vi "Launcher.vi"() -> ()   [LabVIEW 2018]
uses:
  MQTT_Server_Actor/MQTT_Server_Actor.lvclass
  D:/Program Files (x86)/National Instruments/LabVIEW 2018/vi.lib/ActorFramework/Actor/Actor.lvclass
  MQTT_Client_Actor.lvclass
  CreateClient.ctl
  <vilib>/ActorFramework/Actor/Actor.lvclass
  MQTT_Server_Actor Messages/1_StartStopServer Msg/1_StartStopServer Msg.lvclass
  MQTT_Client_Actor Messages/1_CreateClient Msg/1_CreateClient Msg.lvclass
panel:
  in  "ClientNO.":i32=2
  in  "ServerNO.":i32=1
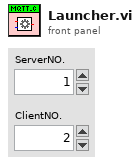
[diagram p1: front panel]
types:
  T1 = typedef "MQTT_Client_Actor.lvlib/MQTT_Client_Actor.lvclass/CreateClient.ctl" = cluster{"address":string, "port":u16, "UserName":string, "Pwd":string}
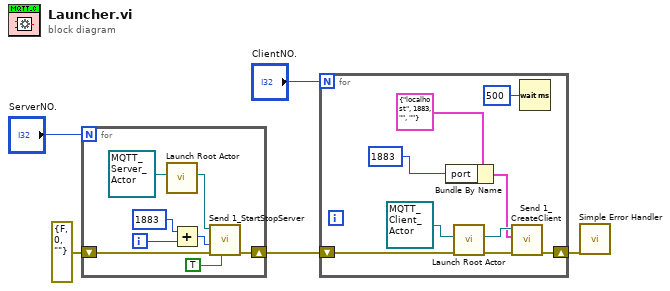
[diagram p0: block diagram]
diagram:
  n1 = for {
    N: "ServerNO." -> [_]
    shift-right: [w8] -> w3
    shift-left: errorcluster {"status"=FALSE, "code"=0, "source"=""} ("error out") -> [w7]
    i -> [w10]
    n2 = call <vilib>:"Launch Root Actor.vi"("Actor"=refnum<class "MQTT_Server_Actor.lvclass"> refnum ("MQTT_Server_Actor.lvlib:MQTT_Server_Actor.lvclass")) -> ("Actor's Enqueuer"=w12:refnum<class "Message Enqueuer.lvclass">)  [unwired: 9 in, 1 out]
    n3 = Add(x=u16 1883 ("remote port (80)"), y=w10) -> (x+y=w9:i32)
    n4 = call "Send 1_StartStopServer.vi"("T:start"=TRUE, "error in (no error)"=w7, "remote port (80)"=w9, "Message Enqueuer in"=w12) -> ("error out"=w8:errorcluster)  [unwired: 6 in, 1 out]
  }
  n5 = for {
    N: "ClientNO." -> [_]
    shift-right: [w15] -> w1
    shift-left: w3 -> [w17]
    n6 = Bundle By Name(cluster=T1 {"address"="localhost", "port"=1883, "UserName"="", "Pwd"=""} ("Create"), "port"=u16 1883 ("remote port (80)")) -> (w19:T1)
    n7 = call <vilib>:"Launch Root Actor.vi"("error in (no error)"=w17, "Actor"=refnum<class "MQTT_Client_Actor.lvclass"> refnum ("MQTT_Client_Actor.lvlib:MQTT_Client_Actor.lvclass")) -> ("error out"=w16:errorcluster, "Actor's Enqueuer"=w21:refnum<class "Message Enqueuer.lvclass">)  [unwired: 8 in]
    n8 = call "Send 1_CreateClient.vi"("error in (no error)"=w16, "Create"=w19, "Message Enqueuer in"=w21) -> ("error out"=w15:errorcluster)  [unwired: 7 in, 1 out]
    n9 = Wait (ms)(milliseconds to wait=u32 500 ("等待时间（毫秒）")) -> ()  [unwired: 1 out]
  }
  n10 = call <vilib>:"Simple Error Handler.vi"("error in (no error)"=w1) -> ()  [unwired: 4 in, 5 out]
